vi "Flavour Descriptor.vi"(10 "Descriptor":string, 11 "Output Actor Hardware in":refnum<class "Output Actor Hardware.lvclass">) -> (2 "Flavoured Descriptor":string, 3 "Output Actor Hardware out":refnum<class "Output Actor Hardware.lvclass">)   [LabVIEW 2015, in "Output Actor Hardware.lvclass"]
uses:
  Output Actor Hardware.lvclass
  Output Actor Hardware.lvclass/Output Actor Hardware.ctl
  Output Actor/Output Actor.lvclass
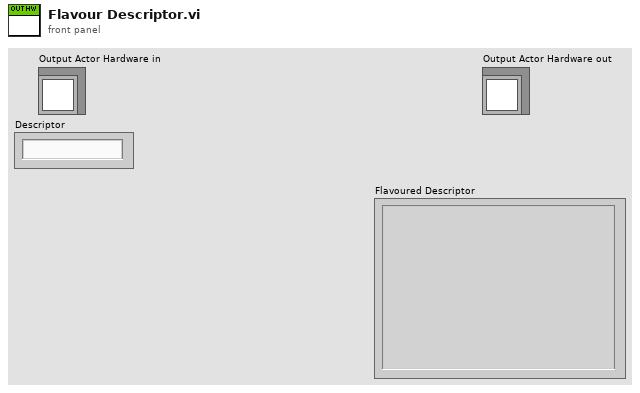
[diagram p1: front panel]
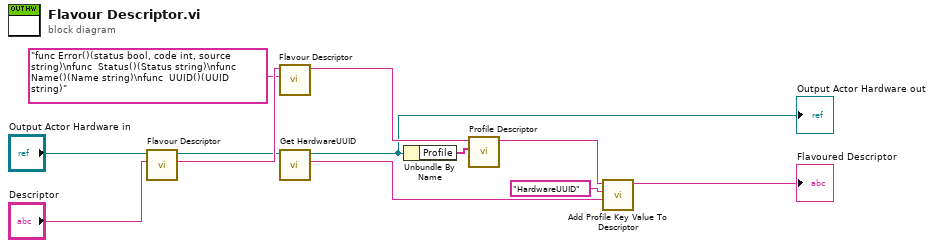
[diagram p0: block diagram]
diagram:
  n1 = call-parent "Flavour Descriptor.vi"("Descriptor"="Descriptor", "output_actor in"="Output Actor Hardware in") -> ("Flavoured Descriptor"=w10:string, "output_actor out"=w3:refnum<class "Output Actor Hardware.lvclass">)  [unwired: 8 in]
  n2 = call "Flavour Descriptor.vi"("Flavour"="func Error()(status bool, code int, source string)\nfunc  Status()(Status string)\nfunc  Name()(Name string)\nfunc  UUID()(UUID string)" ("string"), "Descriptor"=w10) -> ("Flavoured Descriptor"=w7:string)  [unwired: 9 in]
  n3 = call "Get HardwareUUID.vi"("Output Actor Hardware in"=w3) -> ("UUID"=w1:string, "Output Actor Hardware out"=w2:refnum<class "Output Actor Hardware.lvclass">)  [unwired: 8 in, 1 out]
  "Output Actor Hardware out" <- w2
  n4 = Unbundle By Name(w2) -> ("Profile"=w8:string[])
  n5 = call "Profile Descriptor.vi"("Profile"=w8, "Descriptor"=w7) -> ("Flavoured Descriptor"=w6:string)  [unwired: 9 in]
  n6 = call "Add Profile Key Value To Descriptor.vi"("Value"=w1, "Key"="HardwareUUID", "Descriptor"=w6) -> ("Flavoured Descriptor"=→"Flavoured Descriptor":string)  [unwired: 8 in]
